vi "Reset.vi"(8 "error in (no error)":errorcluster, 11 "VISA resource name":refnum<visa-resource-name>) -> (0 "error out":errorcluster, 3 "VISA resource name out":refnum<visa-resource-name>)   [LabVIEW 2015, in "Fluke 289.lvlib"]
doc: "Resets the instrument and then sends a set of default setup commands to the instrument.\n\nNote:\nThis VI will delay 10 seconds to wait the instrument restart."
uses:
  <instrlib>/Fluke 289/Fluke 289.lvlib
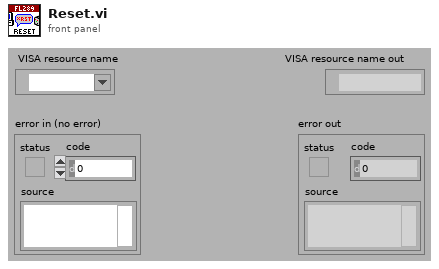
[diagram p1: front panel]
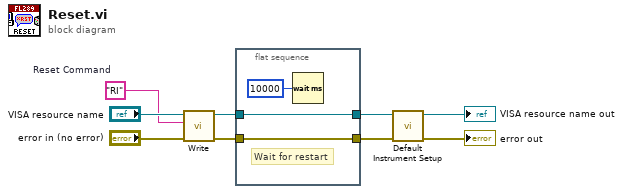
[diagram p0: block diagram]
diagram:
  w7 = "RI"  # Reset Command
  n1 = call <instrlib>:"Write.vi"("error in (no error)"="error in (no error)", "Write Buffer"=w7, "VISA resource name"="VISA resource name") -> ("error out"=w6:errorcluster, "VISA resource name out"=w5:refnum<visa-resource-name>)  [unwired: 7 in]
  n2 = flat-sequence {
    tunnel: w5 -> [w11]
    tunnel: w6 -> [w10]
    tunnel: [w11] -> w2
    tunnel: [w10] -> w1
    frame #0 {
      # "Wait for restart"
      n3 = Wait (ms)(milliseconds to wait=u32 10000) -> ()  [unwired: 1 out]
    }
  }
  n4 = call <instrlib>:"Default Instrument Setup.vi"("error in (no error)"=w1, "VISA resource name"=w2) -> ("error out"=→"error out":errorcluster, "VISA resource name out"=→"VISA resource name out":refnum<visa-resource-name>)  [unwired: 8 in]
